vi "LockinDAQ.setSampling.vi"(6 "AI Buffer Size (S)":i32=100, 8 "error in (no error)":errorcluster, 9 "Sample Mode":T1=10178 items=["Finite Samples"=10178, "Continuous Samples"=10123], 10 "Sampling":T2={"Fs"=204789.0, "#s"=15753}, 11 "LockinDAQ":refnum<class "LockinDAQ.lvclass">) -> (0 "error out":errorcluster, 3 "LockinDAQ out":refnum<class "LockinDAQ.lvclass">)   [LabVIEW 2016, in "LockinDAQ.lvclass"]
doc: "---------------------------------------------------------------\nJKI State Machine Objects™\nhttp://jki.net/state-machine-objects/\nCopyright (C) 2005-2015, JKI <info@jki.net>\nALL RIGHTS RESERVEDJKI State Machine Objects (SMO) 1.0.0.4\nJKI - JKI\nCopyright (c) 2015, JKI"
uses:
  LockinDAQ.lvclass
  Typedefs/Sampling.ctl
  Typedefs/Sample Mode--Ring.ctl
  Typedefs/PrivateEvents--LockinDAQ.setSampling.ctl
  LockinDAQ.lvclass/LockinDAQ.ctl
panel:
  # "For instructions on how to use the JKI State Machine Objects, examples and video tutorials, visit:\nhttp://jki.net/state-machine-objects/\n\nJKI State Machine Objects™\nhttp://jki.net/state-machine-objects/\nCopyright (C) 2005-2015, JKI <info@jki.net>\nALL RIGHTS RESERVED"
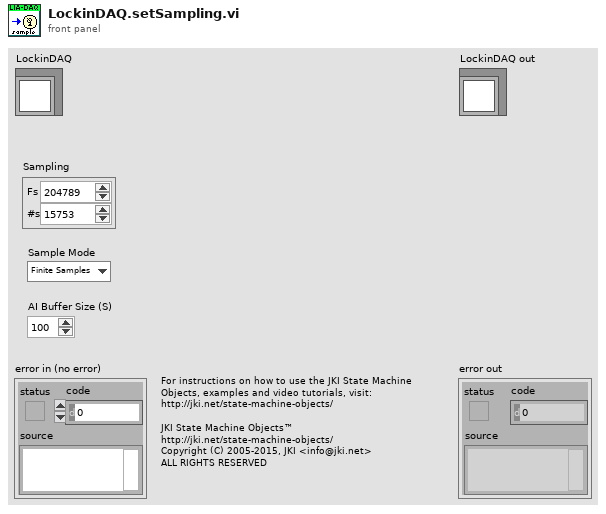
[diagram p1: front panel]
types:
  T1 = typedef "LockinDAQ.lvclass/Sample Mode--Ring.ctl" = i32
  T2 = typedef "LockinDAQ.lvclass/Sampling.ctl" = cluster{"Fs":dbl, "#s":i32}
  T3 = typedef "LockinDAQ.lvclass/PrivateEvents--LockinDAQ.setSampling.ctl" = cluster{"Sampling":T2, "Sample Mode":T1, "AI Buffer Size (S)":i32}
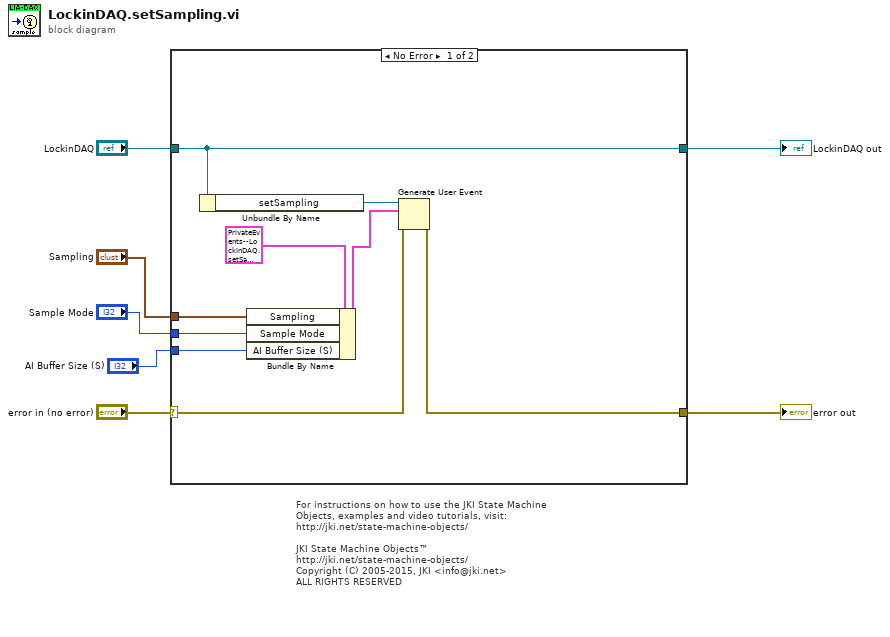
[diagram p0: block diagram]
diagram:
  # "For instructions on how to use the JKI State Machine Objects, examples and video tutorials, visit:\nhttp://jki.net/state-machine-objects/\n\nJKI State Machine Objects™\nhttp://jki.net/state-machine-objects/\nCopyright (C) 2005-2015, JKI <info@jki.net>\nALL RIGHTS RESERVED"
  n1 = case shown="No Error" "error in (no error)" {
    selector: "error in (no error)" -> [w16 w18]
    tunnel: [w14 w18] -> w6
    tunnel: [w13 w17] -> w7
    tunnel: "LockinDAQ" -> [w13 w17]
    tunnel: "Sampling" -> [w10 _]
    tunnel: "Sample Mode" -> [w9 _]
    tunnel: "AI Buffer Size (S)" -> [w8 _]
    frame No Error {
      n2 = Unbundle By Name(w13) -> ("setSampling"=w15:refnum<user-event>)
      n3 = Bundle By Name(cluster=T3 {"Sampling"={"Fs"=204789.0, "#s"=15753}, "Sample Mode"=10178, "AI Buffer Size (S)"=100} ("setSampling"), "Sampling"=w10, "Sample Mode"=w9, "AI Buffer Size (S)"=w8) -> (w11:T3)
      n4 = Generate User Event(user event=w15, event data cluster=w11, error in=w16) -> (error out=w14:errorcluster)  [unwired: 1 in, 1 out]
    }
    frame Error {
    }
  }
  "error out" <- w6
  "LockinDAQ out" <- w7
